vi "Serial Transmit Receive Test.vi"(6 "ready for output":bool, 7 "transfer length":u8=32, 8 "force stop":bool, 9 "input valid":bool, 10 "start transfer":bool, 11 "sample in":u32) -> (0 "data":bool, 1 "output valid":bool, 2 "clk":bool, 3 "sample out":u32, 4 "ready for input":bool)   [LabVIEW 2013]
uses:
  <vilib>/Platform/TimedLoop/XDataNode/timing_clust.ctl
  <vilib>/Platform/TimedLoop/XDataNode/nitl_modes.ctl
  <vilib>/Platform/TimedLoop/XDataNode/wakeup.ctl
  <vilib>/rvi/Emulation/niFpgaSctlEmulationGetInTimedLoop.vi
  <vilib>/rvi/Emulation/niFpgaEmulationReportErrorSimple.vi
  <vilib>/rvi/Emulation/niFpgaGetClockAttributes.vi
  <vilib>/rvi/Emulation/niFpgaCriticalErrorInLSC.vi
  <vilib>/Platform/TimedLoop/XDataNode/XDataNode.xnode
  <vilib>/Platform/TimedLoop/XDataNode/XDNodeRunTimeDep.lvlib
  Source/I2S-TDM.lvlib
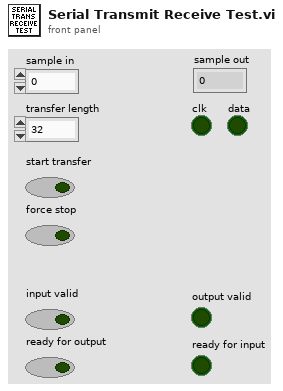
[diagram p1: front panel]
types:
  T1 = typedef "XDNodeRunTimeDep.lvlib/timing_clust.ctl" = cluster{"Expected End [f-1]":u64, "Actual End [f-1]":u64, "Finished Late? [f-1]":bool, "Expected End [i-1]":u64, "Actual End [i-1]":u64, "Finished Late? [i-1]":bool, "Expected Start [i]":u64, "Actual Start [i]":u64, "Expected Start [f]":u64, "Actual Start [f]":u64, "Source Name":string, "Structure Name":string, "Period":i64, "Deadline":i64, "Offset":i64, "Start":i64, "Priority":i32, "Timeout":i32, "Mode":T2, "Wakeup Reason":T3, "Error":errorcluster, "Source Type":string, "Secondary Source Type":string, "Global End Time":u64, "Global Start Time":u64, "Frame Duration":u64, "Iteration Duration":u64, "Assigned CPU":i32, "I/O Scan Engine Mode":u32}
  T2 = typedef "XDNodeRunTimeDep.lvlib/nitl_modes.ctl" = enum32{"No Change", "Process missed periods, maintain original phase", "Discard missed periods, maintain original phase", "Process missed periods, ignore original phase", "Discard missed periods, ignore original phase"}
  T3 = typedef "XDNodeRunTimeDep.lvlib/wakeup.ctl" = enum32{"Normal", "Aborted", "Asynchronous wakeup", "Timing source error", "Timed loop error", "Timeout"}
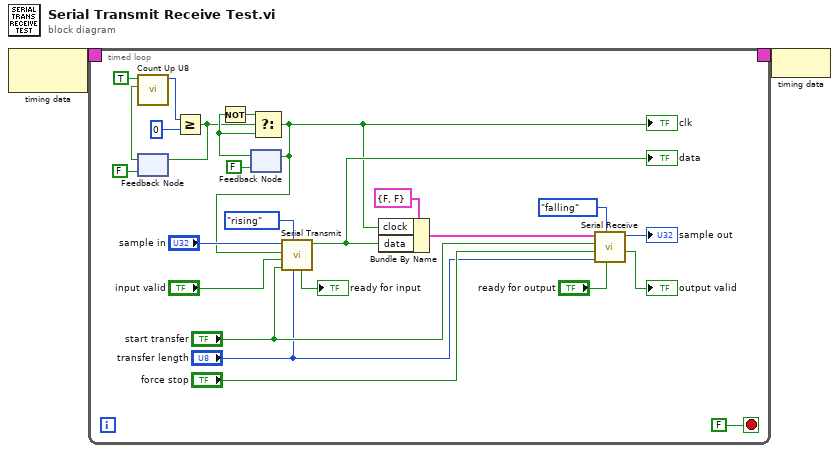
[diagram p0: block diagram]
diagram:
  n1 = node-c288() -> (w2:T1)  [unwired: 1 in]
  n2 = timed-loop {
    timing: w2 -> [_]
    timing-out: [_] -> w1
    stop <- FALSE stop-if-true
    n3 = feedback #1(FALSE) -> (w12:bool)
    n4 = call "Count Up U8.vi"("reset (F)"=w12, "increment"=TRUE) -> ("count"=w10:u8)  [unwired: 9 in]
    n5 = Greater Or Equal?(x=w10, y=u8 0) -> (x >= y?=w7:bool)
    n6 = feedback-in #1(w7) -> ()
    n7 = feedback #2(FALSE) -> (w8:bool)
    n8 = Not(x=w8) -> (.not. x?=w14:bool)
    n9 = Select(t=w14, s=w7, f=w8) -> (s? t:f=w5:bool)
    "clk" <- w5
    n10 = feedback-in #2(w5) -> ()
    n11 = call "Serial Transmit.vi"("transfer length"="transfer length", "serial clock shift edge (falling)"=enum16{"rising", "falling"}."rising", "transmit"="start transfer", "input valid"="input valid", "serial clock in"=w5, "sample"="sample in") -> ("data bit out"=w16:bool, "ready for input"=→"ready for input":bool)  [unwired: 4 in]
    "data" <- w16
    n12 = Bundle By Name(cluster=cluster{"clock":bool, "data":bool} {"clock"=FALSE, "data"=FALSE} ("signals in"), "clock"=w5, "data"=w16) -> (w21:cluster{"clock":bool, "data":bool})
    n13 = call "Serial Receive.vi"("ready for output"="ready for output", "data sampling edge"=enum16{"rising", "falling"}."falling" ("clock sampling edge"), "transfer length"="transfer length", "force stop (F)"="force stop", "start transfer"="start transfer", "signals in"=w21) -> ("output valid"=→"output valid":bool, "sample out"=→"sample out":u32)  [unwired: 3 in, 1 out]
  }
  n14 = node-c288(w1) -> ()
